vi "Start Data Acquisition.vi"(8 "error in (no error)":errorcluster, 11 "Cluster":T1) -> (0 "error out":errorcluster, 2 "data":waveform(dbl)[](array[waveform]), 3 "Cluster 2":T1)   [LabVIEW 2013]
uses:
  <vilib>/DAQmx/read.llb/DAQmx Read (Analog 1D Wfm NChan NSamp).vi
  <vilib>/DAQmx/configure/trigger.llb/DAQmx Start Trigger (Digital Edge).vi
  <vilib>/DAQmx/miscellaneous.llb/DAQmx Fill In Error Info.vi
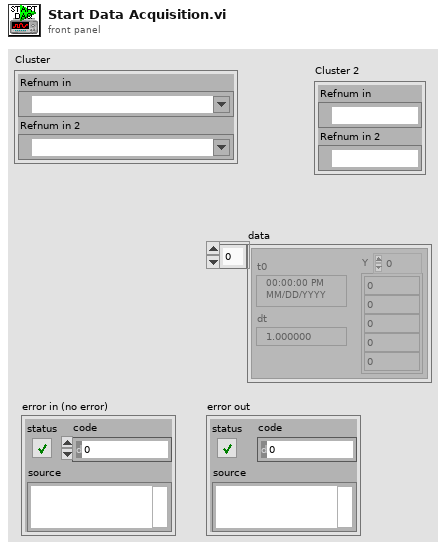
[diagram p1: front panel]
types:
  T1 = cluster{"Refnum in":refnum<k21>, "Refnum in 2":refnum<k21>}
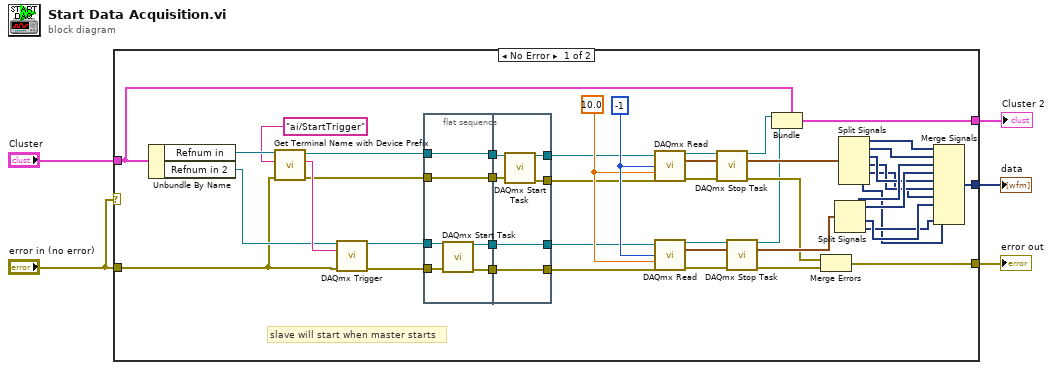
[diagram p0: block diagram]
diagram:
  n1 = case shown="No Error" "error in (no error)" {
    tunnel: [w44 _] -> w5
    tunnel: "Cluster" -> [w43 _]
    tunnel: [w40 w61] -> w3
    tunnel: [w27 _] -> w2
    tunnel: "error in (no error)" -> [w15 w61]
    frame No Error {
      w42 = -1 ("number of samples")
      w41 = 10.0 ("timeout (s)")
      # "slave will start when master starts"
      n2 = Unbundle By Name(w43) -> ("Refnum in"=w18:refnum<k21>, "Refnum in 2"=w16:refnum<k21>)
      n3 = call "Get Terminal Name with Device Prefix.vi"("error in (no error)"=w15, "Local Terminal Name"="ai/StartTrigger", "task/channels in"=w18) -> ("error out"=w10:errorcluster, "Terminal Name with Device Prefix"=w17:tag, "task out"=w13:refnum<k21>)  [unwired: 6 in]
      n4 = call-poly <vilib>:"DAQmx Trigger.vi"("task/channels in"=w16, "source"=w17, "error in"=w15) -> ("task out"=w9:refnum<k21>, "error out"=w7:errorcluster)  [unwired: 11 in]
      n5 = flat-sequence {
        tunnel: [w54] -> w48
        tunnel: w13 -> [w54]
        tunnel: w10 -> [w53]
        tunnel: [w53] -> w47
        tunnel: w9 -> [w52]
        tunnel: [w51] -> w46
        tunnel: w7 -> [w50]
        tunnel: [w49] -> w45
        tunnel: w48 -> [w60]
        tunnel: [w59] -> w12
        tunnel: [w58] -> w11
        tunnel: w47 -> [w57]
        tunnel: [w56] -> w8
        tunnel: w46 -> [w56]
        tunnel: [w55] -> w6
        tunnel: w45 -> [w55]
        frame #0 {
          n6 = call <vilib>:"DAQmx Start Task.vi"("task/channels in"=w52, "error in"=w50) -> ("task out"=w51:refnum<k21>, "error out"=w49:errorcluster)  [unwired: 12 in]
        }
        frame #1 {
          n7 = call <vilib>:"DAQmx Start Task.vi"("task/channels in"=w60, "error in"=w57) -> ("task out"=w59:refnum<k21>, "error out"=w58:errorcluster)  [unwired: 12 in]
        }
      }
      n8 = call-poly <vilib>:"DAQmx Read.vi"("task/channels in"=w12, "number of samples per channel"=w42, "timeout"=w41, "error in"=w11) -> ("task out"=w26:refnum<k21>, "data"=w39:waveform(dbl)[], "error out"=w24:errorcluster)  [unwired: 9 in]
      n9 = call-poly <vilib>:"DAQmx Read.vi"("task/channels in"=w8, "number of samples per channel"=w42, "timeout"=w41, "error in"=w6) -> ("task out"=w22:refnum<k21>, "data"=w38:waveform(dbl)[], "error out"=w20:errorcluster)  [unwired: 9 in]
      n10 = call <vilib>:"DAQmx Stop Task.vi"("task/channels in"=w26, "error in"=w24) -> ("task out"=w25:refnum<k21>, "error out"=w23:errorcluster)  [unwired: 12 in]
      n11 = call <vilib>:"DAQmx Stop Task.vi"("task/channels in"=w22, "error in"=w20) -> ("task out"=w21:refnum<k21>, "error out"=w19:errorcluster)  [unwired: 12 in]
      n12 = Bundle(cluster=w43, "Refnum in"=w25, "Refnum in 2"=w21) -> (w44:T1)
      n13 = Merge Errors(w23, w19) -> (w40:errorcluster)
      n14 = Split Signals(w38) -> (w35:dynamicdata, w34:dynamicdata, w30:dynamicdata, w29:dynamicdata)  [unwired: 4 in]
      n15 = Split Signals(w39) -> (w37:dynamicdata, w36:dynamicdata, w33:dynamicdata, w32:dynamicdata, w31:dynamicdata, w28:dynamicdata)  [unwired: 6 in]
      n16 = Merge Signals(w37, w36, w35, w34, w33, w32, w31, w30, w29, w28) -> (w27:dynamicdata)
    }
    frame Error {
    }
  }
  "data" <- w2
  "error out" <- w3
  "Cluster 2" <- w5
